vi "Vision Testing.vi"() -> ()   [LabVIEW 2018]
uses:
  <vilib>/vision/NI_Vision_Development_Module.lvlib
panel:
  out "Particle Reports (Pixels)":T1(array[cluster]) {"Orientation" format="%.2f"; "Dimensions"."Height" format="%.2f"; "Dimensions"."Width" format="%.2f"; "Center of Mass"."Y" format="%.2f"; "Center of Mass"."X" format="%.2f"; "Bounding Rect"."Bottom" format="%.2f"; "Bounding Rect"."Right" format="%.2f"; "Bounding Rect"."Top" format="%.2f"; "Bounding Rect"."Left" format="%.2f"; "Number of Holes" format="%.2f"; "Area" format="%.2f"}
  out "New Image":T2(plugin-control)
  in  "Color Scheme":T3={"Red or Hue Range"={"Lower value"=0, "Upper value"=255}, "Green or Sat Rabge"={"Lower value"=0, "Upper value"=255}, "Blue or Lua Range"={"Lower value"=0, "Upper value"=255}}
  out "Image Size":cluster{"X Resolution":i32, "Y Resolution":i32}
  out "Original Image":T2(plugin-control)
  in  "File Path":path
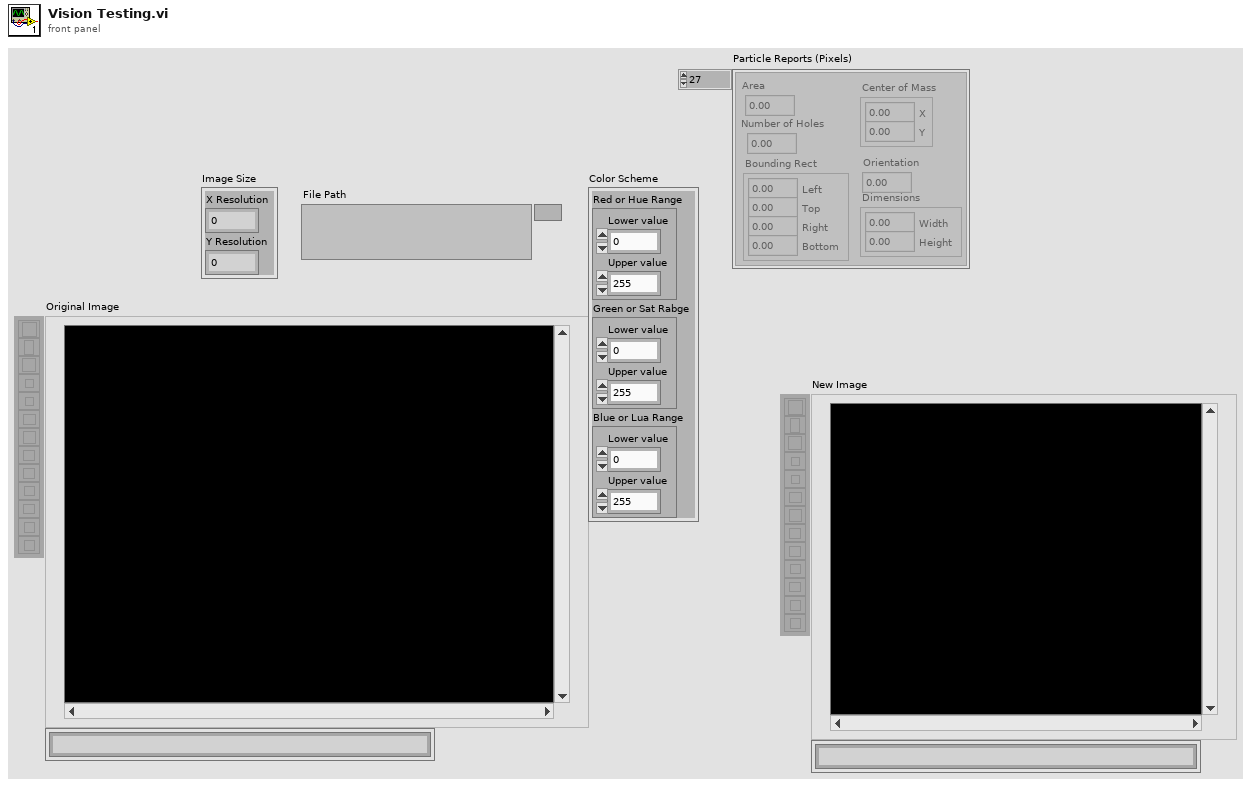
[diagram p1: front panel]
types:
  T1 = cluster{"Area":dbl, "Number of Holes":dbl, "Bounding Rect":cluster{"Left":dbl, "Top":dbl, "Right":dbl, "Bottom":dbl}, "Center of Mass":cluster{"X":dbl, "Y":dbl}, "Orientation":dbl, "Dimensions":cluster{"Width":dbl, "Height":dbl}}[]
  T2 = typedef "IMAQ Image.ctl" = refnum<image>
  T3 = cluster{"Red or Hue Range":cluster{"Lower value":i32, "Upper value":i32}, "Green or Sat Rabge":cluster{"Lower value":i32, "Upper value":i32}, "Blue or Lua Range":cluster{"Lower value":i32, "Upper value":i32}}
  T4 = typedef "Image Type" = u32
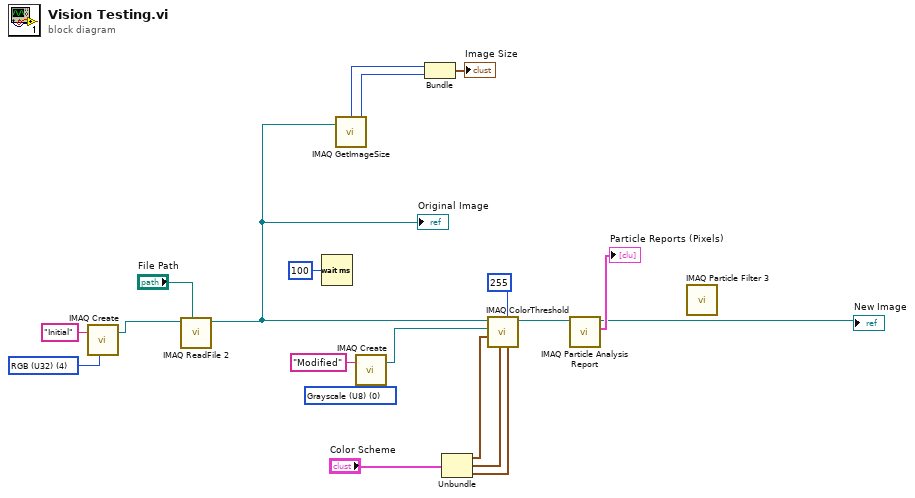
[diagram p0: block diagram]
diagram:
  w12 = T4 0 items=["Grayscale (U8)", "Grayscale (I16)", "Grayscale (SGL)", "Complex (CSG)", "RGB (U32)", "HSL (U32)", "RGB (U64)", "Grayscale (U16)"] ("Image Type")
  w20 = T4 4 items=["Grayscale (U8)", "Grayscale (I16)", "Grayscale (SGL)", "Complex (CSG)", "RGB (U32)", "HSL (U32)", "RGB (U64)", "Grayscale (U16)"] ("Image Type")
  n1 = call "IMAQ Create"("Image Name"="Initial", "Image Type"=w20) -> ("New Image"=w17:T2)  [unwired: 3 in, 1 out]
  n2 = call "IMAQ ReadFile 2"("File Path"="File Path", "Image"=w17) -> ("Image Out"=w10:T2)  [unwired: 5 in, 4 out]
  "Original Image" <- w10
  n3 = Wait (ms)(milliseconds to wait=u32 100) -> ()  [unwired: 1 out]
  n4 = call "IMAQ GetImageSize"("Image"=w10) -> ("Y Resolution"=w16:i32, "X Resolution"=w15:i32)  [unwired: 3 in, 1 out]
  n5 = call "IMAQ Create"("Image Name"="Modified", "Image Type"=w12) -> ("New Image"=w9:T2)  [unwired: 3 in, 1 out]
  n6 = Bundle("X Resolution"=w15, "Y Resolution"=w16) -> (→"Image Size":cluster{"X Resolution":i32, "Y Resolution":i32})  [unwired: 1 in]
  n7 = Unbundle("Color Scheme") -> ("Red or Hue Range"=w7:cluster{"Lower value":i32, "Upper value":i32}, "Green or Sat Rabge"=w6:cluster{"Lower value":i32, "Upper value":i32}, "Blue or Lua Range"=w5:cluster{"Lower value":i32, "Upper value":i32})
  n8 = call "IMAQ ColorThreshold"("Blue or Luma or Val or Inten Range"=w5, "Replace Value"=255, "Green or Sat Range"=w6, "Red or Hue Range"=w7, "Image Dst"=w9, "Image Src"=w10) -> ("Image Dst Out"=w4:T2)  [unwired: 4 in, 1 out]
  n9 = call "IMAQ Particle Analysis Report"("Image"=w4) -> ("Particle Reports (Pixels)"=→"Particle Reports (Pixels)":T1, "Image Out (duplicate)"=→"New Image":T2)  [unwired: 5 in, 4 out]
  n10 = call "IMAQ Particle Filter 3"() -> ()  [unwired: 13 in, 3 out]
